vi "HFRR ADV v09 new software.vi"() -> ()   [LabVIEW 2025] (continued)
              n274 = Close Reference(reference=w377, error in (no error)=w378) -> (error out=w375:errorcluster)
            }
            n275 = Close Reference(reference=w367, error in (no error)=w368) -> (error out=w366:errorcluster)
            n276 = Close Reference(reference=w365, error in (no error)=w366) -> (error out=w360:errorcluster)
            "error out 7" <- w360
            n277 = call <vilib>:"Clear Errors.vi"("error in (no error)"=w360) -> ("error out"=w359:errorcluster)  [unwired: 5 in, 1 out]
            n278 = local write "Service Password enable"(FALSE ("Service Password enable")) -> ()
            n279 = call <userlib>:"Fit VI window to Largest Dec.vi"("error in (no error)"=w359, "border spacing (2 px)"=1) -> ("error out"=w364:errorcluster, "dup VI Ref"=w362:refnum<vi>)  [unwired: 4 in]
            n280 = invoke on="Invoke Node" class="VI" method="FP.Run-Time Position.Maximized"(reference=w362, error in=w364) -> (error out=w363:errorcluster)  [unwired: 2 in, 3 out]
            n281 = call <vilib>:"Clear Errors.vi"("error in (no error)"=w363) -> ()  [unwired: 5 in, 2 out]
          }
          frame True {
          }
        }
      }
      event "Heater Button": Value Change {
        n282 = event-data() -> ()  [unwired: 1 in, 6 out]
        n283 = local read "Heater Button"() -> (w381:bool)
        n284 = case shown="True" w381 {
          frame True {
            n285 = stacked-sequence {
              frame #0 {
                n286 = Wait (ms)(milliseconds to wait=u32 1500) -> ()  [unwired: 1 out]
              }
              frame #1 {
                n287 = local read "Set Temp"() -> (w383:dbl)
                n288 = Number To Fractional String(number=w383, precision (6)=i16 2) -> (F-format string=w386:string)  [unwired: 2 in]
                n289 = Concatenate Strings("ST;" ("Command"), w386) -> (w385:string)
                n290 = local write "Command"(w385) -> ()
              }
              frame #2 {
                n291 = Wait (ms)(milliseconds to wait=u32 1500) -> ()  [unwired: 1 out]
              }
              frame #3 {
                n292 = local write "Command"("HE;1" ("Command")) -> ()
              }
              frame #4 {
                n293 = Wait (ms)(milliseconds to wait=u32 1500) -> ()  [unwired: 1 out]
              }
            }
          }
          frame False {
            n294 = stacked-sequence {
              frame #0 {
                n295 = Wait (ms)(milliseconds to wait=u32 1500) -> ()  [unwired: 1 out]
              }
              frame #1 {
                n296 = Concatenate Strings("ST;" ("Command"), "0" ("string")) -> (w393:string)
                n297 = local write "Command"(w393) -> ()
              }
              frame #2 {
                n298 = Wait (ms)(milliseconds to wait=u32 1500) -> ()  [unwired: 1 out]
              }
              frame #3 {
                n299 = local write "Command"("HE;0" ("Command")) -> ()
              }
              frame #4 {
                n300 = Wait (ms)(milliseconds to wait=u32 1500) -> ()  [unwired: 1 out]
              }
            }
          }
        }
      }
      event "Headen Service Button": Value Change {
        n301 = event-data() -> ()  [unwired: 1 in, 6 out]
        n302 = local read "Headen Service Button"() -> (w398:bool)
        n303 = case shown="True" w398 {
          frame False {
            n304 = property on="Password 3" class="Clust (strict)"("Visible"=FALSE) -> ()  [unwired: 2 in, 2 out]
            n305 = property on="Service Password Log" class="Str"("Visible"=FALSE) -> ()  [unwired: 2 in, 2 out]
          }
          frame True {
            n306 = property on="Password 3" class="Clust (strict)"("Visible"=TRUE) -> ()  [unwired: 2 in, 2 out]
            n307 = property on="Service Password Log" class="Str"("Visible"=TRUE) -> ()  [unwired: 2 in, 2 out]
          }
        }
      }
      event "Password 3.Service Password": Value Change {
        n308 = event-data() -> ()  [unwired: 1 in, 6 out]
        n309 = Unbundle By Name("Password 3") -> ("Service Password"=w405:string)
        n310 = call <vilib>:"Trim Whitespace.vi"("string"=w405) -> ("trimmed string"=w403:string)  [unwired: 1 in]
        n311 = Equal?(x=w403, y="Service@123") -> (x = y?=w404:bool)
        n312 = case shown="False" w404 {
          selector: w404 -> [w409 w411]
          frame False {
            n313 = local write "Service Password enable"(w409) -> ()
            n314 = property on="Service Password Log" class="Str"("Visible"=TRUE) -> ()  [unwired: 2 in, 2 out]
            n315 = property on="Tab Control 5" class="TabCtl (strict)"("Tabs Visible?"=TRUE ("Page Labels Display Visible?")) -> ()  [unwired: 2 in, 2 out]
          }
          frame True {
            n316 = property on="Service Password Log" class="Str"("Visible"=FALSE) -> ()  [unwired: 2 in, 2 out]
            "Service Password enable" <- w411
          }
        }
      }
      event "Sign In": Value Change {
        w413 = FALSE ("Visible")
        n317 = event-data() -> ()  [unwired: 1 in, 6 out]
        n318 = property on="About" class="Clust (strict)"("Visible"=w413) -> ()  [unwired: 2 in, 2 out]
        n319 = property on="Password 3" class="Clust (strict)"("Visible"=w413) -> ()  [unwired: 2 in, 2 out]
        n320 = property on="Service Password Log" class="Str"("Visible"=FALSE) -> ()  [unwired: 2 in, 2 out]
      }
      event "Info": Value Change {
        n321 = event-data() -> ()  [unwired: 1 in, 6 out]
        n322 = local read "Info"() -> (w415:bool)
        n323 = case shown="False" w415 {
          frame False {
            n324 = property on="About" class="Clust (strict)"("Visible"=FALSE) -> ()  [unwired: 2 in, 2 out]
          }
          frame True {
            n325 = property on="About" class="Clust (strict)"("Visible"=TRUE) -> ()  [unwired: 2 in, 2 out]
          }
        }
      }
      event "Calibration": Value Change {
        n326 = event-data() -> ()  [unwired: 1 in, 6 out]
        n327 = local read "Calibration"() -> (w419:bool)
        n328 = case shown="False" w419 {
          frame False {
            n329 = property on="Calibration 2" class="TabCtl (strict)"("Visible"=FALSE) -> ()  [unwired: 2 in, 2 out]
            n330 = local write "Cal Password"("" ("Cal Password")) -> ()
          }
          frame True {
            n331 = property on="Calibration 2" class="TabCtl (strict)"("Visible"=TRUE) -> ()  [unwired: 2 in, 2 out]
            n332 = local write "Cal Password"("" ("Cal Password")) -> ()
          }
        }
        n333 = property on="Wrong Password" class="Str"("Visible"=FALSE) -> ()  [unwired: 2 in, 2 out]
      }
      event "Cal Password": Value Change {
        n334 = event-data() -> ()  [unwired: 1 in, 6 out]
        n335 = local read "Cal Password"() -> (w427:string)
        n336 = call <vilib>:"Trim Whitespace.vi"("string"=w427) -> ("trimmed string"=w426:string)  [unwired: 1 in]
        n337 = Equal?(x=w426, y="Cal@321") -> (x = y?=w424:bool)
        n338 = case shown="True" w424 {
          frame False {
            n339 = property on="Wrong Password" class="Str"("Visible"=TRUE) -> ()  [unwired: 2 in, 2 out]
          }
          frame True {
            n340 = property on="Wrong Password" class="Str"("Visible"=FALSE) -> ()  [unwired: 2 in, 2 out]
            n341 = local write "Main Tab"(T2."About" ("Main Tab")) -> ()
            n342 = local write "Cal Password"("" ("Cal Password")) -> ()
            n343 = local write "Main Dashboard Buttons"(T1."About" ("Main Dashboard Buttons")) -> ()
            n344 = local write "Tab Control 5"(T11."Temperature Calibration" ("Tab Control 5")) -> ()
            n345 = property on="Calibration 2" class="TabCtl (strict)"("Visible"=FALSE) -> ()  [unwired: 2 in, 2 out]
            n346 = property on="Tab Control 5" class="TabCtl (strict)"("Tabs Visible?"=FALSE ("Page Labels Display Visible?")) -> ()  [unwired: 2 in, 2 out]
            n347 = local write "Calibration"(FALSE ("Calibration")) -> ()
          }
        }
      }
      event "Calibration Selection": Value Change {
        n348 = event-data() -> ()  [unwired: 1 in, 6 out]
        n349 = local read "Calibration Selection"() -> (w438:T8)
        n350 = case shown="Default" w438 {
          tunnel: [T7."Stroke" ("Main Calibration Tab") T7."Friction" ("Main Calibration Tab") T7."Main" ("Main Calibration Tab") T7."Temperature" ("Main Calibration Tab")] -> w437
          frame "Stroke Calibration" {
          }
          frame "Friction Force Calibration" {
          }
          frame Default {
          }
          frame "Temperature Calibration" {
          }
        }
        n351 = local write "Main Calibration Tab"(w437) -> ()
      }
      event "Quit": Value Change {
        n352 = event-data() -> ()  [unwired: 1 in, 6 out]
      }
    }
    n353 = Wait (ms)(milliseconds to wait=u32 100) -> ()  [unwired: 1 out]
  }
  n354 = local write "Auto stop temp"(w14) -> ()
  n355 = while {
    stop <- w445 stop-if-true
    n356 = Wait (ms)(milliseconds to wait=u32 200) -> ()  [unwired: 1 out]
    n357 = local read "Quit"() -> (w445:bool)
  }
  n358 = local write "main tab sub"(enum32{"Page 1", "Page 2"}."Page 1" ("main tab sub")) -> ()
  n359 = local write "USERNAME"(w31) -> ()
  n360 = local write "Main Tab"(T2."HOME" ("Main Tab")) -> ()
  n361 = local write "USER ID"(w31) -> ()
  n362 = property on="Auto Scar Check  2" class="Clust (strict)"("Visible"=w14) -> (error out=w17:errorcluster)  [unwired: 2 in, 1 out]
  n363 = property on="Quit" class="Bool (strict)"("Value"=FALSE ("Quit")) -> (error out=w33:errorcluster)  [unwired: 2 in, 1 out]
  n364 = while {
    shift-right: [w447] -> _
    shift-left: "Enum - Selector" -> [w448]
    stop <- w449 stop-if-true
    # "Auto Start Logic Loop"
    n365 = case shown="\"Maintain Stage\"" w448 {
      tunnel: [w452 w458 w470 w502 w533 Auto_Start_enum."Exit" ("Enum - Selector") Auto_Start_enum."Init" ("Enum - Selector")] -> w447
      frame "Init", Default {
        n366 = local read "Auto Start Test"() -> (w451:bool)
        n367 = Select(t=Auto_Start_enum."Humidity & Temperature On" ("Enum - Selector"), s=w451, f=Auto_Start_enum."Init") -> (s? t:f=w452:T14)
      }
      frame "Humidity & Temperature On" {
        n368 = flat-sequence {
          tunnel: [Auto_Start_enum."Reach point" ("Enum - Selector")] -> w455
          frame #0 {
            w460 = T17."Disabled and Grayed Out" ("Disabled")
            w461 = TRUE ("Heater Button")
            n369 = property on="Humidity" class="Bool (strict)"("DisabledEnum"=w460) -> ()  [unwired: 2 in, 2 out]
            n370 = property on="Heater Button" class="Bool (strict)"("DisabledEnum"=w460) -> ()  [unwired: 2 in, 2 out]
            n371 = local write "Heater Button"(w461) -> ()
            n372 = local write "Humidity"(w461) -> ()
            n373 = property on="Heater Button" class="Bool (strict)"("Val(Sgnl)"=TRUE ("Value (Signaling)")) -> ()  [unwired: 2 in, 2 out]
          }
          frame #1 {
            n374 = Wait (ms)(milliseconds to wait=u32 3000) -> ()  [unwired: 1 out]
          }
          frame #2 {
            w463 = TRUE ("Reach point temp")
            n375 = local write "Reach point Humidity"(w463) -> ()
            n376 = local write "Reach point temp"(w463) -> ()
          }
        }
        n377 = local read "Auto Start Test"() -> (w457:bool)
        n378 = Not(x=w457) -> (.not. x?=w456:bool)
        n379 = Select(t=Auto_Start_enum."close", s=w456, f=w455) -> (s? t:f=w458:T14)
      }
      frame "Reach point" {
        w471 = TRUE ("PAUSE")
        w479 = 1.0 ("y")
        w482 = 1.0 ("y")
        n380 = local read "Set Temperature:"() -> (w483:dbl)
        n381 = local read "Set Humidity:"() -> (w478:dbl)
        n382 = local read "Humidity ( %RH )"() -> (w484:dbl)
        n383 = Add(x=w483, y=w482) -> (x+y=w481:dbl)
        n384 = Subtract(x=w483, y=w482) -> (x-y=w480:dbl)
        n385 = Add(x=w478, y=w479) -> (x+y=w477:dbl)
        n386 = Subtract(x=w478, y=w479) -> (x-y=w476:dbl)
        n387 = local read "TEMP"() -> (w485:dbl)
        n388 = In Range and Coerce(upper limit=w477, x=w484, lower limit=w476) -> (In Range?=w465:bool)  [unwired: 1 out]
        n389 = In Range and Coerce(upper limit=w481, x=w485, lower limit=w480) -> (In Range?=w466:bool)  [unwired: 1 out]
        n390 = case shown="True" w465 {
          frame False {
          }
          frame True {
            n391 = case shown="True" "Reach point Humidity" {
              selector: "Reach point Humidity" -> [_ w491]
              frame False {
              }
              frame True {
                n392 = local read "EVENT LOG"() -> (w488:string)
                n393 = Not(x=w491) -> (.not. x?=w490:bool)
                n394 = local write "Reach point Humidity"(w490) -> ()
                n395 = call "Event Log.vi"("Content"="Target Humidity reached", "EVENT LOG"=w488) -> ("EVENT LOG"=w489:string)  [unwired: 8 in, 1 out]
                n396 = local write "EVENT LOG"(w489) -> ()
              }
            }
          }
        }
        n397 = case shown="True" w466 {
          frame False {
          }
          frame True {
            n398 = case shown="True" "Reach point temp" {
              selector: "Reach point temp" -> [_ w497]
              frame False {
              }
              frame True {
                n399 = local read "EVENT LOG"() -> (w494:string)
                n400 = Not(x=w497) -> (.not. x?=w496:bool)
                n401 = local write "Reach point temp"(w496) -> ()
                n402 = call "Event Log.vi"("Content"="Target Temperature reached", "EVENT LOG"=w494) -> ("EVENT LOG"=w495:string)  [unwired: 8 in, 1 out]
                n403 = local write "EVENT LOG"(w495) -> ()
              }
            }
          }
        }
        n404 = local read "Auto Start Test"() -> (w469:bool)
        n405 = And(x=w466, y=w465) -> (x .and. y?=w475:bool)
        n406 = Select(t=Auto_Start_enum."Maintain Stage" ("Enum - Selector"), s=w475, f=Auto_Start_enum."Reach point" ("Enum - Selector")) -> (s? t:f=w472:T14)
        n407 = Not(x=w469) -> (.not. x?=w468:bool)
        n408 = Select(t=Auto_Start_enum."close", s=w468, f=w472) -> (s? t:f=w470:T14)
        n409 = call "ELAPSED TIMER VI.vi"("RESET"=w471, "PAUSE"=w471) -> ()  [unwired: 7 in, 3 out]
      }
      frame "Maintain Stage" {
        w511 = 2.0 ("y")
        w510 = 1.0 ("y")
        # "Humidity and  temperatures Set Point  have been reached"
        n410 = local read "Set Temperature:"() -> (w517:dbl)
        n411 = local read "Set Humidity:"() -> (w514:dbl)
        n412 = local read "Humidity ( %RH )"() -> (w518:dbl)
        n413 = Add(x=w517, y=w510) -> (x+y=w516:dbl)
        n414 = Subtract(x=w517, y=w510) -> (x-y=w515:dbl)
        n415 = local read "TEMP"() -> (w519:dbl)
        n416 = Add(x=w514, y=w511) -> (x+y=w513:dbl)
        n417 = Subtract(x=w514, y=w511) -> (x-y=w512:dbl)
        n418 = In Range and Coerce(upper limit=w516, x=w519, lower limit=w515) -> (In Range?=w509:bool)  [unwired: 1 out]
        n419 = In Range and Coerce(upper limit=w513, x=w518, lower limit=w512) -> (In Range?=w508:bool)  [unwired: 1 out]
        n420 = And(x=w509, y=w508) -> (x .and. y?=w507:bool)
        n421 = Not(x=w507) -> (.not. x?=w506:bool)
        n422 = call "ELAPSED TIMER VI.vi"("TARGET"=60.0, "RESET"=w506, "PAUSE"=FALSE) -> ("ELAPSED INDICATION"=w503:bool)  [unwired: 6 in, 2 out]
        n423 = case shown="True" w503 {
          tunnel: w503 -> [_ w522]
          tunnel: [Auto_Start_enum."Maintain Stage" ("Enum - Selector") w521] -> w501
          frame False {
          }
          frame True {
            n424 = stacked-sequence {
              tunnel: w522 -> [_ _ _ _ _]
              tunnel: [_ _ _ _ Auto_Start_enum."Start Stage" ("Enum - Selector")] -> w521
              frame #0 {
                n425 = local read "EVENT LOG"() -> (w524:string)
                n426 = call "Event Log.vi"("Content"="Humidity and temperature set point has stabilized.", "EVENT LOG"=w524) -> ("EVENT LOG"=w525:string)  [unwired: 8 in, 1 out]
                n427 = local write "EVENT LOG"(w525) -> ()
              }
              frame #1 {
                n428 = Wait (ms)(milliseconds to wait=u32 100) -> ()  [unwired: 1 out]
              }
              frame #2 {
                n429 = local read "EVENT LOG"() -> (w528:string)
                n430 = call "Event Log.vi"("Content"="Auto Test Started", "EVENT LOG"=w528) -> ("EVENT LOG"=w529:string)  [unwired: 8 in, 1 out]
                n431 = local write "EVENT LOG"(w529) -> ()
              }
              frame #3 {
                w530 = TRUE ("RUN")
                n432 = local write "RUN"(w530) -> ()
                "Auto Start Temp" <- w530
              }
              frame #4 {
              }
            }
          }
        }
        n433 = local read "Auto Start Test"() -> (w500:bool)
        n434 = Not(x=w500) -> (.not. x?=w499:bool)
        n435 = Select(t=Auto_Start_enum."close", s=w499, f=w501) -> (s? t:f=w502:T14)
      }
      frame "Start Stage" {
        w532 = TRUE ("PAUSE")
        n436 = local read "Auto Start Test"() -> (w537:bool)
        n437 = Not(x=w537) -> (.not. x?=w536:bool)
        n438 = Select(t=Auto_Start_enum."close" ("Enum - Selector"), s=w536, f=Auto_Start_enum."Start Stage" ("Enum - Selector")) -> (s? t:f=w533:T14)
        n439 = call "ELAPSED TIMER VI.vi"("RESET"=w532, "PAUSE"=w532) -> ()  [unwired: 7 in, 3 out]
      }
      frame "close" {
        w539 = FALSE ("Heater Button")
        n440 = local write "RUN"(w539) -> ()
        n441 = local write "Heater Button"(w539) -> ()
        n442 = local write "Humidity"(w539) -> ()
        n443 = local write "Auto Start Test"(w539) -> ()
        n444 = property on="Heater Button" class="Bool (strict)"("Val(Sgnl)"=FALSE ("Value (Signaling)")) -> ()  [unwired: 2 in, 2 out]
      }
      frame "Exit" {
      }
    }
    n445 = Wait (ms)(milliseconds to wait=u32 100) -> ()  [unwired: 1 out]
    n446 = local read "Quit"() -> (w449:bool)
  }
  n447 = property on="Service Password Log" class="Str"("Visible"=w14) -> ()  [unwired: 2 in, 2 out]
  n448 = property on="Password 3" class="Clust (strict)"("Visible"=w14) -> ()  [unwired: 2 in, 2 out]
  n449 = while {
    stop <- w568 stop-if-true
    w551 = errorcluster {"status"=FALSE, "code"=0, "source"=""} ("error in (no error) 3")
    # "this loop is for manual report generation"
    n450 = local read "Confirm Measrurement"() -> (w550:bool)
    n451 = case shown="True" w550 {
      selector: w550 -> [_ w658]
      tunnel: errorcluster {"status"=FALSE, "code"=0, "source"=""} ("error in (no error) 3") -> [_ w659]
      tunnel: [_ w657] -> _
      frame False {
      }
      frame True {
        n452 = stacked-sequence {
          tunnel: w659 -> [_ w692 _]
          tunnel: w658 -> [_ _ w799]
          tunnel: [_ w680 _] -> w657
          frame #0 {
            n453 = String To Path(string="C:\\LAB-IQ\\Image Calibrate v01.dcf") -> (path=w662:path)
            n454 = Open/Create/Replace File ("Open File")(file path (use dialog)=w662) -> (refnum out=w663:refnum<file>)  [unwired: 5 in, 2 out]
            n455 = for {
              N: 4 -> [_]
              tunnel: w663 -> [w669]
              i -> [w665]
              n456 = Read from Text File ("Read File")(file (use dialog)=w669) -> (text=w670:string)  [unwired: 3 in, 3 out]
              n457 = String Subset(string=w670, offset (0)=6, length (rest)=10 ("length (rest)")) -> (substring=w666:string)
              n458 = Fract/Exp String To Number(string=w666) -> (number=w664:dbl)  [unwired: 3 in, 1 out]
              n459 = case shown="3" w665 {
                tunnel: w664 -> [w671 w672 _ w673 _]
                frame 0 {
                  n460 = local write "5x Gain"(w671) -> ()
                }
                frame 1 {
                  n461 = local write "10x Gain"(w672) -> ()
                }
                frame 2 {
                }
                frame 3 {
                  n462 = local write "100x gain"(w673) -> ()
                }
                frame 4, Default {
                }
              }
            }
          }
          frame #1 {
            n463 = local read "TEST STANDARD"() -> (w675:T3)
            n464 = case shown="\"ISO 12156\"" w675 {
              tunnel: ["ASTM D6079" "ISO 12156"] -> w674
              frame "ASTM D6079", Default {
              }
              frame "ISO 12156" {
              }
            }
            n465 = call "IMAGE ANALYSIS.vi"("Enum"=POST_ANALYSIS_ENUM."GET MEASUREMENTS", "error in"=w692) -> ("error out"=w699:errorcluster)  [unwired: 8 in, 1 out]
            n466 = local read "Magnification :"() -> (w685:string)
            n467 = call "Stall Data Flow.vim"("value in"=w699, "milliseconds to wait"=u32 1000) -> ("value out"=w698:errorcluster)  [unwired: 1 out]
            n468 = local read "Test File List :"() -> (w696:string)
            n469 = case shown="\"10x\"" w685 {
              tunnel: [w735 w736] -> w683
              frame "5x", Default {
                n470 = local read "5x Gain"() -> (w735:dbl)
              }
              frame "10x" {
                # "5x"
                n471 = local read "10x Gain"() -> (w736:dbl)
              }
            }
            n472 = call "IMAGE ANALYSIS.vi"("Enum"=POST_ANALYSIS_ENUM."READ", "error in"=w698) -> ("error out"=w695:errorcluster, "data out"=w686:string)  [unwired: 8 in]
            n473 = Match Pattern(string=w686, regular expression="\"type\": ") -> (after substring=w690:string)  [unwired: 1 in, 3 out]
            n474 = call "IMAGE PATH CREATION PY.vi"("error in (no error)"=w695, "File Name :"=w696) -> ("error out"=w694:errorcluster, "File Path"=w682:path, "File Path String:"=w677:string)  [unwired: 7 in]
            n475 = Match Pattern(string=w690, regular expression=",") -> (before substring=w676:string)  [unwired: 1 in, 3 out]
            n476 = local read "Calibration Tab"() -> (w679:enum32{"Measrument", "Calibrate"})
            n477 = call "Stall Data Flow.vim"("value in"=w694, "milliseconds to wait"=u32 250) -> ("value out"=w678:errorcluster)  [unwired: 1 out]
            n478 = Equal?(x=w676, y="\"rectangle\"") -> (x = y?=w687:bool)
            n479 = case shown="False" w687 {
              tunnel: w686 -> [w741 w796]
              tunnel: w683 -> [_ w787]
              tunnel: cluster{"major":dbl, "minor":dbl, "average":dbl} {"major"=0.0, "minor"=0.0, "average"=0.0} -> [w739 w783]
              tunnel: [w738 w780] -> w681
              tunnel: w676 -> [w740 _]
              tunnel: w683 -> [w737 _]
              frame False {
                n480 = Equal?(x=w740, y="\"line\"") -> (x = y?=w742:bool)
                n481 = case shown="True" w742 {
                  tunnel: w741 -> [_ w757]
                  tunnel: w739 -> [w744 w756]
                  tunnel: [w744 w754] -> w738
                  tunnel: w737 -> [_ w753]
                  frame False {
                  }
                  frame True {
                    w752 = 0.0 ("Major Axis")
                    n482 = Match Pattern(string=w757, regular expression="\"length_px\":") -> (after substring=w755:string)  [unwired: 1 in, 3 out]
                    n483 = property on="Major Axis" class="DigNum (strict)"("Caption.Text"="") -> ()  [unwired: 2 in, 2 out]
                    n484 = property on="Minor Axis" class="DigNum (strict)"("Caption.Text"="") -> ()  [unwired: 2 in, 2 out]
                    n485 = property on="Average" class="DigNum (strict)"("Caption.Text"="Line") -> ()  [unwired: 2 in, 2 out]
                    n486 = Fract/Exp String To Number(string=w755, default (0 dbl)=0.0 ("default (0 DBL)")) -> (number=w751:dbl)  [unwired: 2 in, 1 out]
                    "Pixel Value" <- w751
                    n487 = Multiply(x=w751, y=w753) -> (x*y=w764:dbl)
                    n488 = Multiply(x=w764, y=1000.0) -> (x*y=w747:dbl)
                    n489 = Divide(x=w747, y=1000.0) -> (x/y=w750:dbl)
                    n490 = local write "Measurment (mm)"(w750) -> ()
                    n491 = Bundle By Name(cluster=w756, "average"=w747) -> (w754:cluster{"major":dbl, "minor":dbl, "average":dbl})
                    n492 = Number To Fractional String(number=w747, precision (6)=i16 1) -> (F-format string=w746:string)  [unwired: 2 in]
                    n493 = local write "Minor Axis"(w752) -> ()
                    n494 = local write "Major Axis"(w752) -> ()
                    n495 = Fract/Exp String To Number(string=w746) -> (number=w745:dbl)  [unwired: 3 in, 1 out]
                    n496 = local write "Average"(w745) -> ()
                  }
                }
              }
              frame True {
                w784 = 1000.0 ("y")
                w790 = 0.0 ("default (0 DBL)")
                n497 = Match Pattern(string=w796, regular expression=" \"width_px\":") -> (after substring=w794:string)  [unwired: 1 in, 3 out]
                n498 = Match Pattern(string=w794, regular expression="\"height_px\":") -> (before substring=w792:string, after substring=w791:string)  [unwired: 1 in, 2 out]
                n499 = Fract/Exp String To Number(string=w792, default (0 dbl)=w790) -> (number=w789:dbl)  [unwired: 2 in, 1 out]
                n500 = Fract/Exp String To Number(string=w791, default (0 dbl)=w790) -> (number=w788:dbl)  [unwired: 2 in, 1 out]
                n501 = Multiply(x=w789, y=w787) -> (x*y=w786:dbl)
                n502 = Multiply(x=w788, y=w787) -> (x*y=w785:dbl)
                n503 = Multiply(x=w786, y=w784) -> (x*y=w770:dbl)
                n504 = Multiply(x=w785, y=w784) -> (x*y=w768:dbl)
                n505 = Add(x=w770, y=w768) -> (x+y=w782:dbl)
                n506 = property on="Major Axis" class="DigNum (strict)"("Caption.Text"="Major Axis") -> ()  [unwired: 2 in, 2 out]
                n507 = property on="Minor Axis" class="DigNum (strict)"("Caption.Text"="Minor Axis") -> ()  [unwired: 2 in, 2 out]
                n508 = property on="Average" class="DigNum (strict)"("Caption.Text"="Average") -> ()  [unwired: 2 in, 2 out]
                n509 = Divide(x=w782, y=2.0) -> (x/y=w766:dbl)
                n510 = Bundle By Name(cluster=w783, "major"=w770, "minor"=w768, "average"=w766) -> (w780:cluster{"major":dbl, "minor":dbl, "average":dbl})
                n511 = Number To Fractional String(number=w768, precision (6)=i16 1) -> (F-format string=w775:string)  [unwired: 2 in]
                n512 = Number To Fractional String(number=w766, precision (6)=i16 1) -> (F-format string=w776:string)  [unwired: 2 in]
                n513 = Number To Fractional String(number=w770, precision (6)=i16 1) -> (F-format string=w774:string)  [unwired: 2 in]
                n514 = Fract/Exp String To Number(string=w775) -> (number=w767:dbl)  [unwired: 3 in, 1 out]
                n515 = Fract/Exp String To Number(string=w776) -> (number=w765:dbl)  [unwired: 3 in, 1 out]
                n516 = Fract/Exp String To Number(string=w774) -> (number=w769:dbl)  [unwired: 3 in, 1 out]
                n517 = local write "Major Axis"(w769) -> ()
                n518 = local write "Average"(w765) -> ()
                n519 = local write "Minor Axis"(w767) -> ()
              }
            }
            n520 = case shown="\"Measrument\", Default" w679 {
              tunnel: w682 -> [w709 _]
              tunnel: w681 -> [w708 _]
              tunnel: [w705 w734] -> w680
              tunnel: w678 -> [w707 w734]
              tunnel: w677 -> [w706 _]
              tunnel: w674 -> [w704 _]
              frame "Measrument", Default {
                n521 = stacked-sequence {
                  tunnel: w709 -> [w727 _]
                  tunnel: w708 -> [w725 _]
                  tunnel: w707 -> [w723 _]
                  tunnel: w706 -> [w722 _]
                  tunnel: [w717 _] -> w705
                  tunnel: w704 -> [w710 _]
                  frame #0 {
                    n522 = call "IMAGE ANALYSIS.vi"("Enum"=POST_ANALYSIS_ENUM."SAVE IMAGE", "error in"=w723, "IMAGE FILE PATH"=w722) -> ("error out"=w721:errorcluster)  [unwired: 7 in, 1 out]
                    n523 = call "Stall Data Flow.vim"("value in"=w721, "milliseconds to wait"=u32 1000) -> ("value out"=w712:errorcluster)  [unwired: 1 out]
                    n524 = local read "Test File List :"() -> (w729:string)
                    n525 = call "IMAGE ANALYSIS.vi"("Enum"=POST_ANALYSIS_ENUM."MINIMIZE UI", "error in"=w712) -> ("error out"=w719:errorcluster)  [unwired: 8 in, 1 out]
                    n526 = Bundle By Name(cluster=T24 {"File Name"="", "Test Method"="", "Operator"="", "Fuel Description"="", "Date and time"=""} ("Main Ref"), "Test Method"=w710, "File Name"=w729) -> (w730:T24)
                    n527 = call "Stall Data Flow.vim"("value in"=w719, "milliseconds to wait"=u32 1500) -> ("value out"=w714:errorcluster)  [unwired: 1 out]
                    n528 = call "duf file read.vi"("error in (no error)"=w714, "Main Ref"=w730) -> ("error out"=w728:errorcluster, "Main Ref 2"=w726:T24)  [unwired: 8 in]
                    n529 = call "DETECTION REPORT for manual.vi"("error in (no error)"=w728, "return value 3"=w725, "Image File Path"=w727, "Main Ref"=w726) -> ("error out"=w724:errorcluster)  [unwired: 7 in]
                    n530 = call <vilib>:"Clear Errors.vi"("error in (no error)"=w724) -> ("error out"=w715:errorcluster)  [unwired: 5 in, 1 out]
                    n531 = call "IMAGE ANALYSIS.vi"("Enum"=POST_ANALYSIS_ENUM."MINIMIZE UI", "error in"=w715) -> ("error out"=w717:errorcluster)  [unwired: 8 in, 1 out]
                  }
                  frame #1 {
                    n532 = local write "Main Tab"(T2."HOME" ("Main Tab")) -> ()
                    n533 = local write "Main Dashboard Buttons"(T1."Home" ("Main Dashboard Buttons")) -> ()
                  }
                }
              }
              frame "Calibrate" {
              }
            }
          }
          frame #2 {
            n534 = Not(x=w799) -> (.not. x?=w798:bool)
            n535 = local write "Confirm Measrurement"(w798) -> ()
            n536 = local read "Calibration Tab"() -> (w797:enum32{"Measrument", "Calibrate"})
            n537 = case shown="\"Measrument\", Default" w797 {
              frame "Measrument", Default {
                (unwired) T19."HOME" ("Main Tab")
                n538 = local write "Main Tab"(T2."HOME" ("Main Tab")) -> ()
              }
              frame "Calibrate" {
              }
            }
          }
        }
      }
    }
    n539 = local read "Humidity"() -> (w542:bool)
    n540 = local read "Save Change"() -> (w547:bool)
    n541 = local read "Calibrate"() -> (w548:bool)
    n542 = local read "Auto Start Test"() -> (w543:bool)
    n543 = case shown="True" w548 {
      selector: w548 -> [_ w655]
      frame False {
      }
      frame True {
        n544 = Not(x=w655) -> (.not. x?=w654:bool)
        n545 = local write "Calibrate"(w654) -> ()
        n546 = local write "Calibration Tab"(enum32{"Measrument", "Calibrate"}."Calibrate" ("Calibration Tab")) -> ()
      }
    }
    n547 = case shown="True" w547 {
      selector: w547 -> [_ w599]
      frame False {
      }
      frame True {
        n548 = stacked-sequence {
          tunnel: w599 -> [_ _ _ _ w653]
          frame #0 {
            n549 = call "IMAGE ANALYSIS.vi"("Enum"=POST_ANALYSIS_ENUM."HIDE UI") -> ()  [unwired: 9 in, 2 out]
          }
          frame #1 {
            n550 = local read "100x gain"() -> (w601:dbl)
            n551 = local read "10x Gain"() -> (w602:dbl)
            n552 = local read "5x Gain"() -> (w603:dbl)
            n553 = Number To Fractional String(number=w602, width (-)=i16 4, precision (6)=i16 7) -> (F-format string=w624:string)  [unwired: 1 in]
            n554 = Number To Fractional String(number=0.0, width (-)=i16 4, precision (6)=i16 7) -> (F-format string=w619:string)  [unwired: 1 in]
            n555 = Number To Fractional String(number=w601, width (-)=i16 4, precision (6)=i16 7) -> (F-format string=w607:string)  [unwired: 1 in]
            n556 = Number To Fractional String(number=w603, width (-)=i16 10 ("precision (6)"), precision (6)=i16 7) -> (F-format string=w633:string)  [unwired: 1 in]
            n557 = Concatenate Strings("[CH1]" ("string"), w633, " - 5x Gain" ("string"), "\r") -> (w623:string)
            n558 = Concatenate Strings("[CH2]" ("string"), w624, " - 10x Gain" ("string"), "\r") -> (w622:string)
            n559 = Concatenate Strings("[CH3]" ("string"), w619, " - 20x Gain" ("string"), "\r") -> (w613:string)
            n560 = Concatenate Strings("[CH4]" ("string"), w607, " - 100x Gain" ("string"), "\r") -> (w606:string)
            n561 = String To Path(string="C:\\LAB-IQ\\Image Calibrate v01.dcf") -> (path=w636:path)
            n562 = Concatenate Strings(w623, w622, w613, w606) -> (w621:string)
            n563 = call <vilib>:"Write Characters To File.vi"("append to file? (new file:F)"=FALSE, "character string"=w621, "file path (dialog if empty)"=w636) -> ()  [unwired: 2 in, 1 out]
          }
          frame #2 {
            n564 = String To Path(string="C:\\LAB-IQ\\Image Calibrate v01.dcf") -> (path=w639:path)
            n565 = Open/Create/Replace File ("Open File")(file path (use dialog)=w639) -> (refnum out=w640:refnum<file>)  [unwired: 5 in, 2 out]
            n566 = for {
              N: 4 -> [_]
              tunnel: w640 -> [w646]
              i -> [w642]
              n567 = Read from Text File ("Read File")(file (use dialog)=w646) -> (text=w647:string)  [unwired: 3 in, 3 out]
              n568 = String Subset(string=w647, offset (0)=6, length (rest)=10 ("length (rest)")) -> (substring=w643:string)
              n569 = Fract/Exp String To Number(string=w643) -> (number=w641:dbl)  [unwired: 3 in, 1 out]
              n570 = case shown="3" w642 {
                tunnel: w641 -> [w648 w649 _ w650 _]
                frame 0 {
                  n571 = local write "5x Gain"(w648) -> ()
                }
                frame 1 {
                  n572 = local write "10x Gain"(w649) -> ()
                }
                frame 2 {
                }
                frame 3 {
                  n573 = local write "100x gain"(w650) -> ()
                }
                frame 4, Default {
                }
              }
            }
          }
          frame #3 {
            n574 = call "IMAGE ANALYSIS.vi"("Enum"=POST_ANALYSIS_ENUM."SHOW UI") -> ()  [unwired: 9 in, 2 out]
          }
          frame #4 {
            n575 = Not(x=w653) -> (.not. x?=w652:bool)
            n576 = local write "Save Change"(w652) -> ()
          }
        }
      }
    }
    n577 = case shown="False" w543 {
      tunnel: w542 -> [w569 _]
      frame False {
        n578 = case shown="True" w569 {
          frame False {
          }
          frame True {
            n579 = local read "Set Humidity:"() -> (w573:dbl)
            n580 = local read "Set Humidity:"() -> (w576:dbl)
            n581 = local read "Humidity ( %RH )"() -> (w577:dbl)
            n582 = Subtract(x=w573, y=2.0) -> (x-y=w571:dbl)
            n583 = Add(x=w576, y=2.0) -> (x+y=w572:dbl)
            n584 = In Range and Coerce(upper limit=w572, x=w577, lower limit=w571) -> (In Range?=w570:bool)  [unwired: 1 out]
            n585 = case shown="True" w570 {
              frame False {
              }
              frame True {
                n586 = case shown="False" "Manual Humididty Reached" {
                  selector: "Manual Humididty Reached" -> [_ w580]
                  frame False {
                  }
                  frame True {
                    n587 = Not(x=w580) -> (.not. x?=w579:bool)
                    n588 = local write "Manual Humididty Reached"(w579) -> ()
                    n589 = local read "EVENT LOG"() -> (w582:string)
                    n590 = call "Event Log.vi"("Content"="Target Humidity reached", "EVENT LOG"=w582) -> ("EVENT LOG"=w581:string)  [unwired: 8 in, 1 out]
                    n591 = local write "EVENT LOG"(w581) -> ()
                  }
                }
              }
            }
          }
        }
      }
      frame True {
        n592 = local write "Manual Humididty Reached"(TRUE ("Manual Humididty Reached")) -> ()
      }
    }
    n593 = local read "Cap Live Image"() -> (w563:bool)
    n594 = local read "SCAR MEASURMENT"() -> (w566:enum32{"Auto Scar", "Manual Scar"})
    n595 = Wait (ms)(milliseconds to wait=u32 250) -> ()  [unwired: 1 out]
    n596 = Equal?(x=w566, y=enum32{"Auto Scar", "Manual Scar"}."Manual Scar" ("SCAR MEASURMENT")) -> (x = y?=w564:bool)
    n597 = And(x=w564, y=w563) -> (x .and. y?=w562:bool)
    n598 = case shown="True" w562 {
      selector: w562 -> [_ w878]
      frame False {
      }
      frame True {
        n599 = stacked-sequence {
          tunnel: [_ _ _ w893 _] -> _
          tunnel: w878 -> [_ _ _ _ w900]
          frame #0 {
            w879 = 0.0
            n600 = local write "Major Axis"(w879) -> ()
            n601 = local write "Minor Axis"(w879) -> ()
            n602 = local write "Average"(w879) -> ()
          }
          frame #1 {
            n603 = call "CAMERA LIVE FEED FGV.vi"("Enum - Menu"=CAMERA_LIVE_FEED_ENUM."CAMERA MINIMIZE") -> ()  [unwired: 9 in, 2 out]
          }
          frame #2 {
            n604 = local read "FILE 3"() -> (w887:string)
            n605 = call <vilib>:"Trim Whitespace.vi"("string"="C:\\LAB-IQ\\images\\") -> ("trimmed string"=w889:string)  [unwired: 1 in]
            n606 = String To Path(string=w889) -> (path=w888:path)
            n607 = Concatenate Strings(w887, ".png" ("string")) -> (w886:string)
            n608 = Build Path(base path=w888, name or relative path=w886) -> (appended path=w884:path)
            n609 = Path To String(path=w884) -> (string=w883:string)
            n610 = call "CAMERA LIVE FEED FGV.vi"("Enum - Menu"=CAMERA_LIVE_FEED_ENUM."CAMERA SAVE", "Image Path"=w883) -> ("error out"=w881:errorcluster)  [unwired: 8 in, 1 out]
            n611 = case shown="No Error" w881 {
              frame No Error {
                n612 = One Button Dialog(message="Image saved successfully") -> ()  [unwired: 1 in, 1 out]
              }
              frame Error {
              }
            }
          }
          frame #3 {
            n613 = call "LIST FILE NAMES.vi"() -> ("error out"=w895:errorcluster, "filenames"=w892:string[])  [unwired: 10 in]
            n614 = call "IMAGE ANALYSIS.vi"("Enum"=POST_ANALYSIS_ENUM."SHOW UI", "error in"=w895) -> ("error out"=w893:errorcluster)  [unwired: 8 in, 1 out]
            n615 = property on="Test File List :" class="CmbBox"("Strings[]"=w892) -> ()  [unwired: 2 in, 2 out]
          }
          frame #4 {
            (unwired) T23."Report" ("Main Dashboard Buttons")
            (unwired) T25."Report" ("Main Dashboard Buttons")
            n616 = Not(x=w900) -> (.not. x?=w899:bool)
            n617 = local write "Zoom Factore"(0.0 ("Zoom Factore")) -> ()
            n618 = local write "Cap Live Image"(w899) -> ()
            n619 = local write "Main Tab"(T2."Adv Scar Report" ("Main Tab")) -> ()
            n620 = property on="Cap Live Image" class="Bool (strict)"("BoolText.Text"="Capture Image" ("Boolean Text.Text")) -> ()  [unwired: 2 in, 2 out]
            n621 = local write "Main Dashboard Buttons"(T1."Report" ("Main Dashboard Buttons")) -> ()
          }
        }
      }
    }
    n622 = local read "change Gain"() -> (w546:bool)
    n623 = local read "Back Square"() -> (w545:bool)
    n624 = case shown="True" w546 {
      selector: w546 -> [_ w590]
      frame False {
      }
      frame True {
        n625 = stacked-sequence {
          tunnel: w590 -> [_ w598]
          frame #0 {
            n626 = local read "Actual (µm)"() -> (w594:dbl)
            n627 = local read "Pixel Value"() -> (w593:dbl)
            n628 = local read "Magnification :"() -> (w592:string)
            n629 = Divide(x=w594, y=w593) -> (x/y=w591:dbl)
            n630 = case shown="\"10x\"" w592 {
              tunnel: w591 -> [w595 w596]
              frame "10x" {
                n631 = local write "10x Gain"(w595) -> ()
              }
              frame "5x", Default {
                n632 = local write "5x Gain"(w596) -> ()
              }
            }
          }
          frame #1 {
            n633 = Not(x=w598) -> (.not. x?=w597:bool)
            n634 = local write "change Gain"(w597) -> ()
          }
        }
      }
    }
    n635 = case shown="True" w545 {
      selector: w545 -> [_ w588]
      frame False {
      }
      frame True {
        n636 = Not(x=w588) -> (.not. x?=w587:bool)
        n637 = local write "Back Square"(w587) -> ()
        n638 = local write "Calibration Tab"(enum32{"Measrument", "Calibrate"}."Measrument" ("Calibration Tab")) -> ()
      }
    }
    n639 = local read "Rectangle Tool"() -> (w557:bool)
    n640 = local read "Clear ROI Tool"() -> (w556:bool)
    n641 = local read "Open Image"() -> (w561:bool)
    n642 = local read "line tool"() -> (w558:bool)
    n643 = local read "OUT"() -> (w559:bool)
    n644 = local read "In"() -> (w560:bool)
    n645 = case shown="True" w561 {
      selector: w561 -> [_ w866]
      tunnel: [w862 w868] -> _
      tunnel: w551 -> [w862 w867]
      frame False {
      }
      frame True {
        n646 = Not(x=w866) -> (.not. x?=w865:bool)
        n647 = local write "Open Image"(w865) -> ()
        n648 = call "IMAGE ANALYSIS.vi"("Enum"=POST_ANALYSIS_ENUM."HIDE UI", "error in"=w867) -> ("error out"=w875:errorcluster)  [unwired: 8 in, 1 out]
        n649 = call "File Dialog"("start path"=path "C:/LAB-IQ/images", "error in"=w875) -> ("selected path"=w864:path, "error out"=w873:errorcluster)  [unwired: 10 in, 2 out]
        "Image path  2" <- w864
        n650 = call <vilib>:"Clear Errors.vi"("error in (no error)"=w873) -> ("error out"=w872:errorcluster)  [unwired: 5 in, 1 out]
        n651 = call "IMAGE ANALYSIS.vi"("Enum"=POST_ANALYSIS_ENUM."OPEN FILE", "error in"=w872, "File Path"=w864) -> ("error out"=w871:errorcluster)  [unwired: 7 in, 1 out]
        n652 = call <vilib>:"Clear Errors.vi"("error in (no error)"=w871) -> ("error out"=w870:errorcluster)  [unwired: 5 in, 1 out]
        n653 = call "IMAGE ANALYSIS.vi"("Enum"=POST_ANALYSIS_ENUM."SHOW UI", "error in"=w870) -> ("error out"=w868:errorcluster)  [unwired: 8 in, 1 out]
        n654 = local write "Zoom Factore"(100.0 ("Zoom Factore")) -> ()
      }
    }
    n655 = case shown="True" w559 {
      selector: w559 -> [_ w847]
      tunnel: w551 -> [w844 w852]
      tunnel: [w844 w846] -> _
      frame False {
      }
      frame True {
        n656 = Not(x=w847) -> (.not. x?=w845:bool)
        n657 = local read "Zoom Factore"() -> (w850:dbl)
        n658 = local write "OUT"(w845) -> ()
        n659 = call "IMAGE ANALYSIS.vi"("Enum"=POST_ANALYSIS_ENUM."ZOOM OUT", "error in"=w852) -> ("error out"=w846:errorcluster)  [unwired: 8 in, 1 out]
        n660 = Divide(x=w850, y=1.2) -> (x/y=w848:dbl)
        n661 = local write "Zoom Factore"(w848) -> ()
      }
    }
    n662 = case shown="True" w560 {
      selector: w560 -> [_ w856]
      tunnel: w551 -> [w853 w861]
      tunnel: [w853 w854] -> _
      frame False {
      }
      frame True {
        n663 = Not(x=w856) -> (.not. x?=w855:bool)
        n664 = local read "Zoom Factore"() -> (w859:dbl)
        n665 = local write "In"(w855) -> ()
        n666 = call "IMAGE ANALYSIS.vi"("Enum"=POST_ANALYSIS_ENUM."ZOOM IN", "error in"=w861) -> ("error out"=w854:errorcluster)  [unwired: 8 in, 1 out]
        n667 = Multiply(x=w859, y=1.2) -> (x*y=w857:dbl)
        n668 = local write "Zoom Factore"(w857) -> ()
      }
    }
    n669 = case shown="True" w556 {
      selector: w556 -> [_ w828]
      tunnel: w551 -> [w826 w830]
      tunnel: [w826 w829] -> _
      frame False {
      }
      frame True {
        n670 = Not(x=w828) -> (.not. x?=w827:bool)
        n671 = local write "Clear ROI Tool"(w827) -> ()
        n672 = call "IMAGE ANALYSIS.vi"("Enum"=POST_ANALYSIS_ENUM."CLEAR ROI", "error in"=w830) -> ("error out"=w829:errorcluster)  [unwired: 8 in, 1 out]
      }
    }
    n673 = case shown="True" w558 {
      selector: w558 -> [_ w840]
      tunnel: w551 -> [w838 w843]
      tunnel: [w838 w841] -> _
      frame False {
      }
      frame True {
        n674 = Not(x=w840) -> (.not. x?=w839:bool)
        n675 = local write "line tool"(w839) -> ()
        n676 = call "IMAGE ANALYSIS.vi"("Enum"=POST_ANALYSIS_ENUM."DRAW LINE", "error in"=w843) -> ("error out"=w841:errorcluster)  [unwired: 8 in, 1 out]
      }
    }
    n677 = case shown="True" w557 {
      selector: w557 -> [_ w834]
      tunnel: w551 -> [w832 w836]
      tunnel: [w832 w835] -> _
      frame False {
      }
      frame True {
        n678 = Not(x=w834) -> (.not. x?=w833:bool)
        n679 = local write "Rectangle Tool"(w833) -> ()
        n680 = call "IMAGE ANALYSIS.vi"("Enum"=POST_ANALYSIS_ENUM."DRAW REC", "error in"=w836) -> ("error out"=w835:errorcluster)  [unwired: 8 in, 1 out]
      }
    }
    n681 = local read "SCAR MEASURMENT"() -> (w544:enum32{"Auto Scar", "Manual Scar"})
    n682 = local read "Fit to Screen Tool"() -> (w553:bool)
    n683 = local read "Resize Tool"() -> (w552:bool)
    n684 = case shown="\"Manual Scar\", Default" w544 {
      frame "Auto Scar" {
        n685 = property on="Cap Live Image" class="Bool (strict)"("BoolText.Text"="Report" ("Boolean Text.Text")) -> ()  [unwired: 2 in, 2 out]
      }
      frame "Manual Scar", Default {
        n686 = property on="Cap Live Image" class="Bool (strict)"("BoolText.Text"="Save Image" ("Boolean Text.Text")) -> ()  [unwired: 2 in, 2 out]
      }
    }
    n687 = local read "ROI Color Tool"() -> (w554:bool)
    n688 = local read "Pan Tool"() -> (w555:bool)
    n689 = case shown="True" w555 {
      selector: w555 -> [_ w822]
      tunnel: w551 -> [w820 w824]
      tunnel: [w820 w823] -> _
      frame False {
      }
      frame True {
        n690 = Not(x=w822) -> (.not. x?=w821:bool)
        n691 = call "IMAGE ANALYSIS.vi"("Enum"=POST_ANALYSIS_ENUM."PAN", "error in"=w824) -> ("error out"=w823:errorcluster)  [unwired: 8 in, 1 out]
        n692 = local write "Pan Tool"(w821) -> ()
      }
    }
    n693 = case shown="True" w552 {
      selector: w552 -> [_ w806]
      tunnel: w551 -> [w801 w803]
      tunnel: [w801 w802] -> _
      frame False {
      }
      frame True {
        n694 = Not(x=w806) -> (.not. x?=w805:bool)
        n695 = local write "Resize Tool"(w805) -> ()
        n696 = call "IMAGE ANALYSIS.vi"("Enum"=POST_ANALYSIS_ENUM."RESIZE MODE", "error in"=w803) -> ("error out"=w802:errorcluster)  [unwired: 8 in, 1 out]
      }
    }
    n697 = case shown="True" w553 {
      selector: w553 -> [_ w811]
      tunnel: [w807 w812] -> _
      tunnel: w551 -> [w807 w810]
      frame False {
      }
      frame True {
        n698 = Not(x=w811) -> (.not. x?=w809:bool)
        n699 = local write "Zoom Factore"(100.0 ("Zoom Factore")) -> ()
        n700 = local write "Fit to Screen Tool"(w809) -> ()
        n701 = call "IMAGE ANALYSIS.vi"("Enum"=POST_ANALYSIS_ENUM."FIT", "error in"=w810) -> ("error out"=w812:errorcluster)  [unwired: 8 in, 1 out]
      }
    }
    n702 = case shown="True" w554 {
      selector: w554 -> [_ w817]
      tunnel: [w814 w818] -> _
      tunnel: w551 -> [w814 w815]
      frame False {
      }
      frame True {
        n703 = Not(x=w817) -> (.not. x?=w816:bool)
        n704 = local write "ROI Color Tool"(w816) -> ()
        n705 = call "IMAGE ANALYSIS.vi"("Enum"=POST_ANALYSIS_ENUM."SET ROI COLOR", "error in"=w815) -> ("error out"=w818:errorcluster)  [unwired: 8 in, 1 out]
      }
    }
    n706 = local read "Quit"() -> (w568:bool)
  }
  n707 = while {
    stop <- w902 stop-if-true
    n708 = local read "Image Path"() -> (w905:path)
    n709 = local read "Print 3"() -> (w908:bool)
    n710 = Equal?(x=w905, y=path "") -> (x = y?=w904:bool)
    n711 = Not(x=w904) -> (.not. x?=w903:bool)
    n712 = property on="Print 3" class="Bool (strict)"("Visible"=w903) -> ()  [unwired: 2 in, 2 out]
    n713 = case shown="True" w908 {
      frame False {
        n714 = local write "Rd"(TRUE ("Boolean 7")) -> ()
      }
      frame True {
        n715 = flat-sequence {
          tunnel: [w948] -> w916
          tunnel: [w935] -> w914
          tunnel: [w945] -> w910
          tunnel: w916 -> [w957]
          tunnel: [w957] -> w915
          tunnel: w914 -> [w956]
          tunnel: [w956] -> w913
          tunnel: [w954] -> w912
          tunnel: [w953] -> w911
          tunnel: w910 -> [w953]
          tunnel: w915 -> [w959]
          tunnel: w913 -> [w960]
          tunnel: w912 -> [_]
          tunnel: w911 -> [w958]
          frame #0 {
            n716 = case shown="True" "Rd" {
              frame False {
              }
              frame True {
                n717 = while {
                  tunnel: "abcdefABCDEF" ("string 2") -> [w927]
                  shift-right: [w925] -> w919
                  shift-left: "" -> [w924]
                  i -> [w934]
                  stop <- w933 stop-if-true
                  n718 = Random Number (0-1)() -> (number: 0 to 1=w928:dbl)
                  n719 = Multiply(x=w928, y=62.0) -> (x*y=w930:dbl)
                  n720 = Decrement(x="Length 2") -> (x-1=w923:i16)
                  n721 = To Word Integer(number=w930) -> (16bit integer=w931:i16)
                  n722 = String Subset(string=w927, offset (0)=w931, length (rest)=1 ("length (rest)")) -> (substring=w926:string)
                  n723 = Greater Or Equal?(x=w934, y=w923) -> (x >= y?=w933:bool)
                  n724 = Concatenate Strings(w926, w924) -> (w925:string)
                }
                "String 10" <- w919
                n725 = local write "Rd"(FALSE ("Boolean 7")) -> ()
              }
            }
          }
          frame #1 {
            w946 = "_resized.jpg" ("command line")
            (unwired) ".jpg -resize 320x240 " ("string")
            (unwired) "Choose an Image File" ("prompt")
            # "-resize 1798x425"
            n726 = local read "Image Path"() -> (w940:path)
            n727 = Strip Path(path=w940) -> (stripped path=w935:path, name=w936:string)
            n728 = Match Pattern(string=w936, regular expression=".jpg") -> (before substring=→"before substring 2":string, after substring=→"after substring":string)  [unwired: 1 in, 2 out]
            n729 = Match Pattern(string=w936, regular expression="\\") -> (before substring=w942:string)  [unwired: 1 in, 3 out]
            n730 = Match Pattern(string=w942, regular expression=".jpg") -> (before substring=w941:string)  [unwired: 1 in, 3 out]
            n731 = Concatenate Strings("cmd /c convert " ("string"), w941, ".jpg -resize 320x240  " ("command line"), w941, w946) -> (w949:string)
            n732 = call <vilib>:"System Exec.vi"("run minimized? (F)"=TRUE, "wait until completion? (T)"=TRUE, "working directory"=w935, "command line"=w949) -> ("error out"=w948:errorcluster)  [unwired: 4 in, 3 out]
            "error out 2" <- w948
            n733 = Concatenate Strings(w941, w946) -> (w945:string)
          }
          frame #2 {
            n734 = Wait (ms)(milliseconds to wait=u32 2000 ("millisecond timer value")) -> (millisecond timer value=w954:u32)
          }
          frame #3 {
            n735 = case shown="No Error" w959 {
              tunnel: w960 -> [w963 _]
              tunnel: w958 -> [w961 _]
              frame No Error {
                (unwired) ".jpg" ("string")
                n736 = Path To String(path=w963) -> (string=w967:string)
                n737 = Concatenate Strings(w967, "\\" ("string"), w961) -> (w966:string)
                n738 = String To Path(string=w966) -> (path=w965:path)
                n739 = call <vilib>:"Read JPEG File.vi"("path to JPEG file"=w965) -> ("image data"=w969:T15)  [unwired: 8 in, 2 out]
                "image data" <- w969
                n740 = local write "Print 3"(FALSE ("Print 2")) -> ()
                n741 = call <vilib>:"Draw Flattened Pixmap.vi"("image data"=w969) -> ("new picture"=→"new picture":picture)  [unwired: 8 in]
              }
              frame Error {
              }
            }
          }
        }
      }
    }
    n742 = Wait (ms)(milliseconds to wait=u32 20 ("millisecond timer value")) -> ()  [unwired: 1 out]
    n743 = local read "Quit"() -> (w902:bool)
  }
  n744 = while {
    tunnel: w33 -> [_]
    tunnel: w17 -> [_]
    stop <- w1000 stop-if-true
    # "New Adv Logics"
    n745 = local read "Main Tab"() -> (w980:T2)
    n746 = local read "Main Tab"() -> (w998:T2)
    n747 = local read "Sign In"() -> (w997:bool)
    n748 = case shown="\"Adv Scar\"" w980 {
      frame "HOME", Default {
        n749 = local read "LIVE FEED MIN TEMP"() -> (w1133:bool)
        n750 = local write "LIVE FEED MAX TEMP"(TRUE ("LIVE FEED MAX TEMP")) -> ()
        n751 = local read "CAMERA ROI MIN TEMP"() -> (w1131:bool)
        n752 = case shown="True" w1133 {
          selector: w1133 -> [_ w1140]
          frame False {
          }
          frame True {
            n753 = Not(x=w1140) -> (.not. x?=w1139:bool)
            n754 = local write "LIVE FEED MIN TEMP"(w1139) -> ()
            n755 = call "CAMERA LIVE FEED FGV.vi"("Enum - Menu"=CAMERA_LIVE_FEED_ENUM."CAMERA MINIMIZE") -> ()  [unwired: 9 in, 2 out]
          }
        }
        n756 = case shown="True" w1131 {
          selector: w1131 -> [_ w1137]
          frame False {
          }
          frame True {
            n757 = Not(x=w1137) -> (.not. x?=w1136:bool)
            n758 = local write "CAMERA ROI MIN TEMP"(w1136) -> ()
            n759 = call "IMAGE ANALYSIS.vi"("Enum"=POST_ANALYSIS_ENUM."MINIMIZE UI") -> ()  [unwired: 9 in, 2 out]
          }
        }
        n760 = local write "CAMERA ROI MAX TEMP"(TRUE ("CAMERA ROI MAX TEMP")) -> ()
      }
      frame "Test Setup" {
        n761 = local read "LIVE FEED MIN TEMP"() -> (w1143:bool)
        n762 = local read "CAMERA ROI MIN TEMP"() -> (w1141:bool)
        n763 = local write "LIVE FEED MAX TEMP"(TRUE ("LIVE FEED MAX TEMP")) -> ()
        n764 = case shown="True" w1143 {
          selector: w1143 -> [_ w1150]
          frame False {
          }
          frame True {
            n765 = Not(x=w1150) -> (.not. x?=w1149:bool)
            n766 = local write "LIVE FEED MIN TEMP"(w1149) -> ()
            n767 = call "CAMERA LIVE FEED FGV.vi"("Enum - Menu"=CAMERA_LIVE_FEED_ENUM."CAMERA MINIMIZE") -> ()  [unwired: 9 in, 2 out]
          }
        }
        n768 = case shown="True" w1141 {
          selector: w1141 -> [_ w1147]
          frame False {
          }
          frame True {
            n769 = Not(x=w1147) -> (.not. x?=w1146:bool)
            n770 = local write "CAMERA ROI MIN TEMP"(w1146) -> ()
            n771 = call "IMAGE ANALYSIS.vi"("Enum"=POST_ANALYSIS_ENUM."MINIMIZE UI") -> ()  [unwired: 9 in, 2 out]
          }
        }
        n772 = local write "CAMERA ROI MAX TEMP"(TRUE ("CAMERA ROI MAX TEMP")) -> ()
      }
      frame "Acquire" {
        n773 = local read "LIVE FEED MIN TEMP"() -> (w1153:bool)
        n774 = local write "LIVE FEED MAX TEMP"(TRUE ("LIVE FEED MAX TEMP")) -> ()
        n775 = local read "CAMERA ROI MIN TEMP"() -> (w1151:bool)
        n776 = case shown="True" w1153 {
          selector: w1153 -> [_ w1160]
          frame False {
          }
          frame True {
            n777 = Not(x=w1160) -> (.not. x?=w1159:bool)
            n778 = local write "LIVE FEED MIN TEMP"(w1159) -> ()
            n779 = call "CAMERA LIVE FEED FGV.vi"("Enum - Menu"=CAMERA_LIVE_FEED_ENUM."CAMERA MINIMIZE") -> ()  [unwired: 9 in, 2 out]
          }
        }
        n780 = case shown="True" w1151 {
          selector: w1151 -> [_ w1157]
          frame False {
          }
          frame True {
            n781 = Not(x=w1157) -> (.not. x?=w1156:bool)
            n782 = local write "CAMERA ROI MIN TEMP"(w1156) -> ()
            n783 = call "IMAGE ANALYSIS.vi"("Enum"=POST_ANALYSIS_ENUM."MINIMIZE UI") -> ()  [unwired: 9 in, 2 out]
          }
        }
        n784 = local write "CAMERA ROI MAX TEMP"(TRUE ("CAMERA ROI MAX TEMP")) -> ()
      }
      frame "Adv Scar" {
        n785 = local read "CAMERA ROI MIN TEMP"() -> (w1161:bool)
        n786 = case shown="True" "LIVE FEED MAX TEMP" {
          selector: "LIVE FEED MAX TEMP" -> [_ w1182]
          frame False {
          }
          frame True {
